vi "Set Controller Mode.vi"(8 "error in (no error)":errorcluster, 10 "controller mode":T1=1 items=["Motor Stop", "Positioning-Mode", "Velocity-Mode", "no more action", "set position to reference", "PWM-Mode", "Current-Mode", "Initialize"], 11 "motor slave info in":T2 {"nodeAddr" format="%.0x"}) -> (0 "error out":errorcluster, 2 "valid?":bool, 3 "motor slave info out":T2 {"nodeAddr" format="%.0x"})   [LabVIEW 2017, in "NI_Robotics_KUKA youBot Host.lvlib"]
uses:
  <vilib>/robotics/KUKA youBot/NI_Robotics_KUKA youBot Host.lvlib
  <vilib>/robotics/KUKA youBot/EtherCAT/Motor Slave Info.ctl
  <vilib>/robotics/KUKA youBot/EtherCAT/LowLevel/Mater Handler.ctl
  <vilib>/robotics/KUKA youBot/EtherCAT/Control Mode.ctl
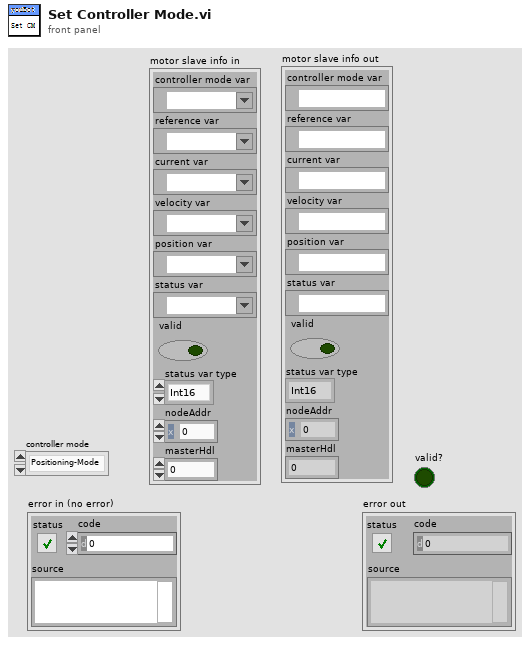
[diagram p1: front panel]
types:
  T1 = typedef "NI_Robotics_KUKA youBot Host.lvlib/Control Mode.ctl" = u8
  T2 = typedef "NI_Robotics_KUKA youBot Host.lvlib/Motor Slave Info.ctl" = cluster{"controller mode var":refnum<k21>, "reference var":refnum<k21>, "current var":refnum<k21>, "velocity var":refnum<k21>, "position var":refnum<k21>, "status var":refnum<k21>, "valid":bool, "status var type":enum16{"Int16", "Int32"}, "nodeAddr":u16, "masterHdl":T3}
  T3 = typedef "NI_Robotics_KUKA youBot Host.lvlib/Mater Handler.ctl" = i32
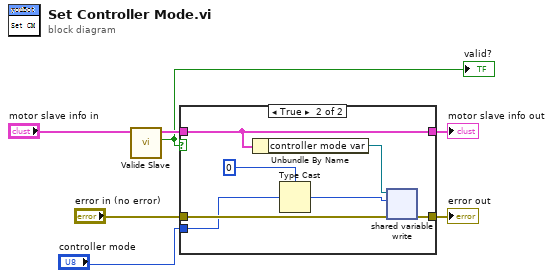
[diagram p0: block diagram]
diagram:
  n1 = call <vilib>:"Valide Slave.vi"("motor slave info in"="motor slave info in") -> ("valid?"=w3:bool, "motor slave info out"=w4:T2)  [unwired: 8 in, 1 out]
  "valid?" <- w3
  n2 = case shown="True" w3 {
    tunnel: [w8 w16] -> w7
    tunnel: "error in (no error)" -> [w8 w15]
    tunnel: "controller mode" -> [_ w14]
    tunnel: w4 -> [w9 w11]
    tunnel: [w9 w11] -> w2
    frame False {
    }
    frame True {
      n3 = Unbundle By Name(w11) -> ("controller mode var"=w10:refnum<k21>)
      n4 = Type Cast(type=u8 0, x=w14) -> (*(type *) &x=w13:u8)
      n5 = shared-variable-write(w10, w15, w13) -> (w16:errorcluster)  [unwired: 1 out]
    }
  }
  "error out" <- w7
  "motor slave info out" <- w2
